vi "test IRIG Deployment.vi"(8 "error in (no error)":errorcluster, 11 "TestCase in":refnum<class "Common System Tests.lvclass">) -> (0 "error out":errorcluster, 3 "TestCase out":refnum<class "Common System Tests.lvclass">)   [LabVIEW 2019, in "Common System Tests.lvclass"]
uses:
  Common System Tests.lvclass
  <vilib>/addons/_JKI Toolkits/VI Tester/TestCase.llb/TestCase.lvclass
  C:/Program Files (x86)/National Instruments/LabVIEW 2019/vi.lib/addons/_JKI Toolkits/VI Tester/TestCase.llb/TestCase.lvclass
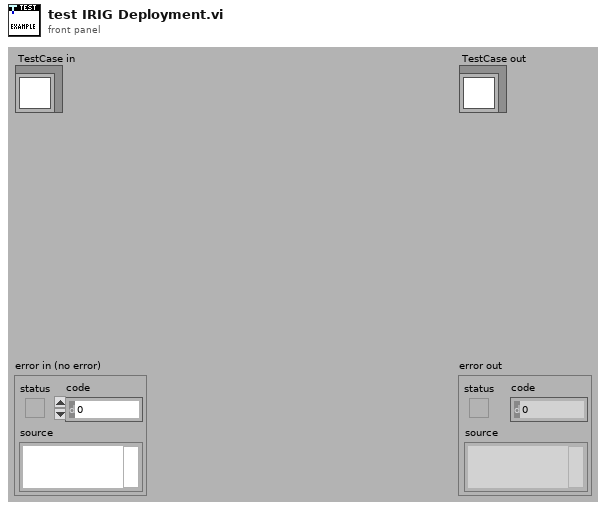
[diagram p1: front panel]
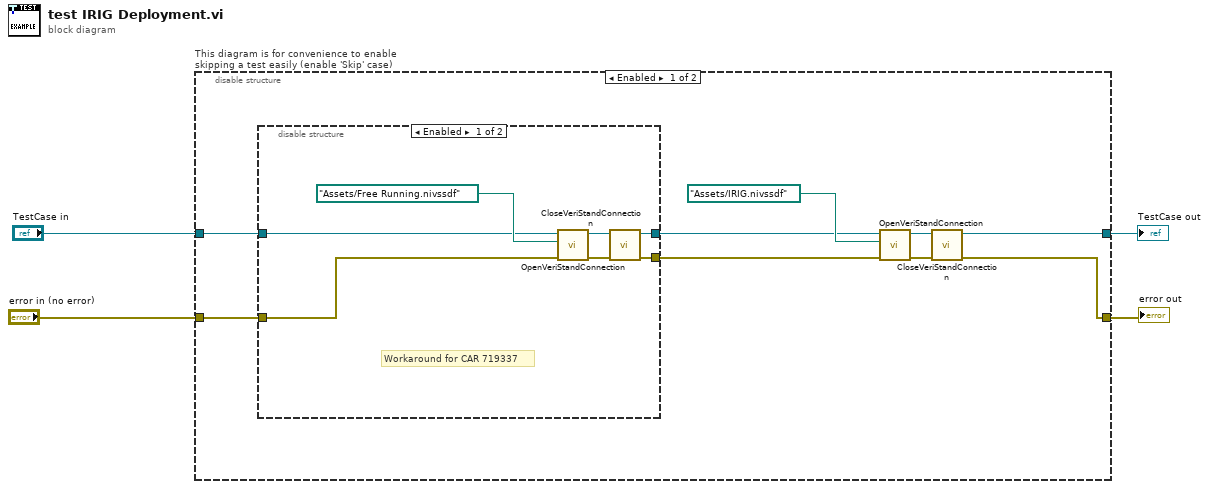
[diagram p0: block diagram]
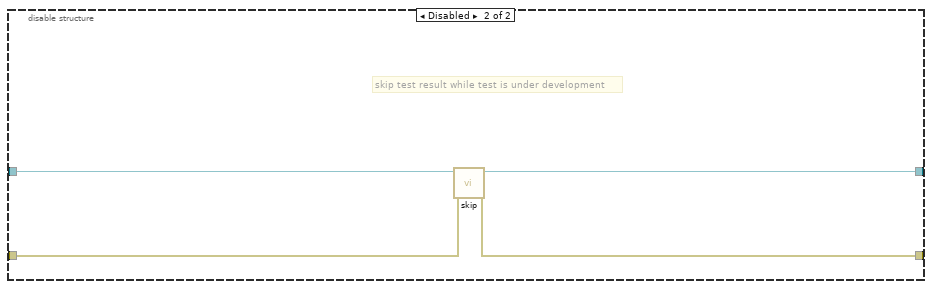
[diagram p3: hidden frame]
diagram:
  n1 = disable-structure "This diagram is for convenience to enable skipping a test easily (enable 'Skip' case)" shown="Enabled" {
    disable-tunnel: "TestCase in" -> [w6 w24]
    disable-tunnel: [w12 w22] -> w1
    disable-tunnel: [w10 w23] -> w3
    disable-tunnel: "error in (no error)" -> [w7 w21]
    frame Enabled {
      n2 = disable-structure shown="Enabled" {
        disable-tunnel: [w17 _] -> w8
        disable-tunnel: w7 -> [w16 _]
        disable-tunnel: w6 -> [w15 _]
        disable-tunnel: [w14 _] -> w5
        frame Enabled {
          # "Workaround for CAR 719337"
          n3 = call-dynamic "OpenVeriStandConnection.vi"("error in (no error)"=w16, "System Definition File"=path "Assets/Free Running.nivssdf", "VeriStand Test Case in"=w15) -> ("error out"=w19:errorcluster, "VeriStand Test Case out"=w20:refnum<class "Common System Tests.lvclass">)  [unwired: 6 in, 1 out]
          n4 = call-dynamic "CloseVeriStandConnection.vi"("error in (no error)"=w19, "VeriStand Test Case in"=w20) -> ("error out"=w17:errorcluster, "VeriStand Test Case out"=w14:refnum<class "Common System Tests.lvclass">)  [unwired: 8 in]
        }
        frame Disabled {
        }
      }
      n5 = call-dynamic "OpenVeriStandConnection.vi"("error in (no error)"=w8, "System Definition File"=path "Assets/IRIG.nivssdf", "VeriStand Test Case in"=w5) -> ("error out"=w11:errorcluster, "VeriStand Test Case out"=w13:refnum<class "Common System Tests.lvclass">)  [unwired: 6 in, 1 out]
      n6 = call-dynamic "CloseVeriStandConnection.vi"("error in (no error)"=w11, "VeriStand Test Case in"=w13) -> ("error out"=w10:errorcluster, "VeriStand Test Case out"=w12:refnum<class "Common System Tests.lvclass">)  [unwired: 8 in]
    }
    frame Disabled {
      # "skip test result while test is under development"
      n7 = call <vilib>:"skip.vi"("error in (no error)"=w21, "TestCase in"=w24) -> ("error out"=w23:errorcluster, "TestCase out"=w22:refnum<class "Common System Tests.lvclass">)  [unwired: 8 in]
    }
  }
  "error out" <- w3
  "TestCase out" <- w1
